vi "BMS Request.vi"(6 "Request":enum16{"Empty", "Load", "Staging"}(ring)=enum."Staging", 8 "error in":errorcluster, 11 "CAN Session In":T1) -> (0 "error out":errorcluster, 3 "CAN Session Out":T1)   [LabVIEW 2016]
uses:
  Program Files (x86)/National Instruments/LabVIEW 2016/examples/robotics/EPOS2 CANOpen Driver/Low Level VIs/Typedefs/CAN Refnum.ctl
  Program Files (x86)/National Instruments/LabVIEW 2016/examples/robotics/EPOS2 CANOpen Driver/Low Level VIs/Typedefs/CAN Session Pointer.ctl
  Program Files (x86)/National Instruments/LabVIEW 2016/examples/robotics/EPOS2 CANOpen Driver/Low Level VIs/Typedefs/CAN Communication References.ctl
  Program Files (x86)/National Instruments/LabVIEW 2016/examples/robotics/EPOS2 CANOpen Driver/Low Level VIs/Typedefs/kill process notifier array.ctl
  Program Files (x86)/National Instruments/LabVIEW 2016/examples/robotics/EPOS2 CANOpen Driver/Low Level VIs/Typedefs/Write Queue.ctl
  Program Files (x86)/National Instruments/LabVIEW 2016/examples/robotics/EPOS2 CANOpen Driver/Low Level VIs/Typedefs/FPGA CAN Frame Cluster.ctl
panel:
  out "appended array":u8[](array[numeric])
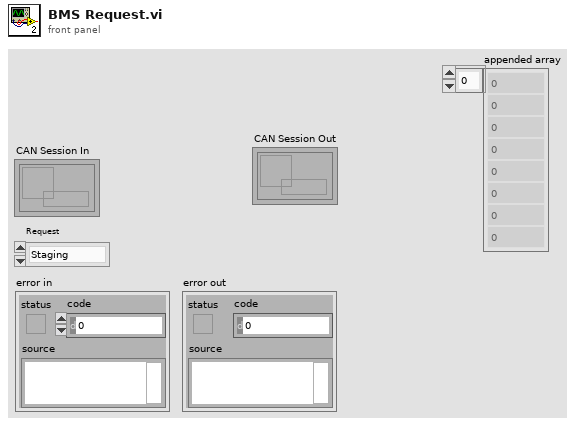
[diagram p1: front panel]
types:
  T1 = typedef "CAN Refnum.ctl" = refnum<k1>
  T2 = typedef "FPGA CAN Frame Cluster.ctl" = cluster{"Timestamp":u64, "Identifier":u32, "Type":u8, "InfoA":u8, "InfoB":u8, "DataLength":u8, "Data":u8[]}
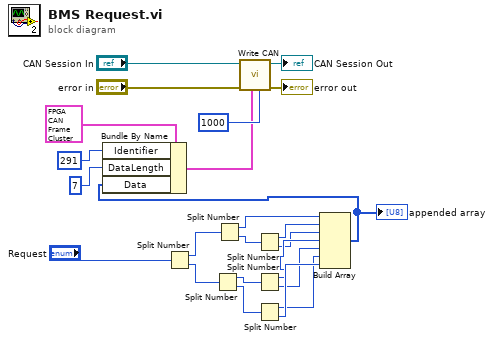
[diagram p0: block diagram]
diagram:
  n1 = Split Number(x="Request") -> (hi(x)=w13:u8, lo(x)=w12:u8)
  n2 = Split Number(x=w12) -> (hi(x)=w10:u8, lo(x)=w9:u8)
  n3 = Split Number(x=w13) -> (hi(x)=w1:u8, lo(x)=w11:u8)
  n4 = Split Number(x=w11) -> (hi(x)=w2:u8, lo(x)=w3:u8)
  n5 = Split Number(x=w10) -> (hi(x)=w4:u8, lo(x)=w5:u8)
  n6 = Split Number(x=w9) -> (hi(x)=w6:u8, lo(x)=w7:u8)
  n7 = Build Array(w1, w2, w3, w4, w5, w6, w7) -> (w8:u8[])
  "appended array" <- w8
  n8 = Bundle By Name(cluster=T2 {"Timestamp"=0, "Identifier"=0, "Type"=0, "InfoA"=0, "InfoB"=0, "DataLength"=0, "Data"=[0, 0, 0, 0, 0, 0, 0, 0]} ("CAN Frame"), "Identifier"=u32 291, "DataLength"=u8 7, "Data"=w8) -> (w19:T2)
  n9 = call "Write CAN.vi"("timeout"=1000, "CAN Frame"=w19, "error in"="error in", "CAN Session In"="CAN Session In") -> ("error out"=→"error out":errorcluster, "CAN Session Out"=→"CAN Session Out":T1)  [unwired: 6 in]
